vi "Music Visualizer Template LV2014.vi"() -> ()   [LabVIEW 2014]
uses:
  <vilib>/sound2/lvsound2.llb/Sampling Mode.ctl
  <vilib>/sound2/lvsound2.llb/Sound File Info (path).vi
  <vilib>/sound2/lvsound2.llb/Sound File Read Open.vi
  <vilib>/sound2/lvsound2.llb/Sound File Read (DBL).vi
  <vilib>/sound2/lvsound2.llb/Sound Output Write (DBL).vi
panel:
  in  "Stop":bool
  in  "Buffer Size (samples)":i32=2048
  in  "Music File":path
  # "Your visualizer here."
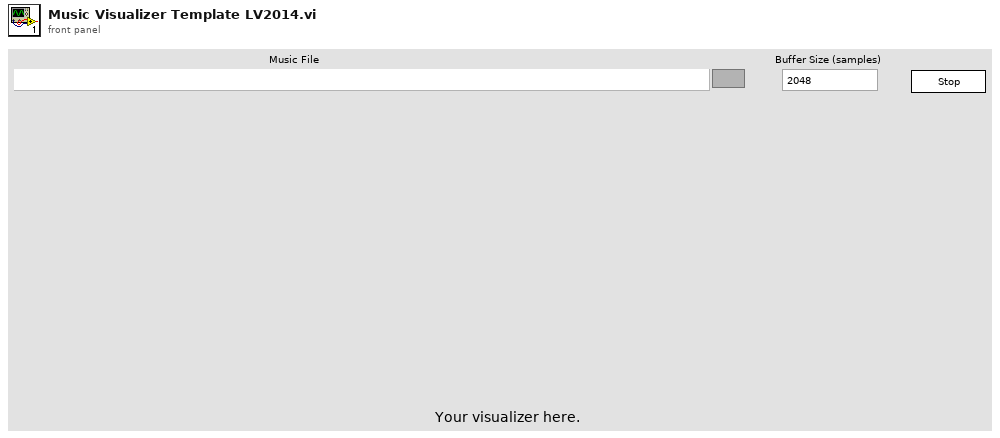
[diagram p1: front panel]
types:
  T1 = typedef "Sampling Mode.ctl" = i32
  T2 = typedef "Sound Data Format.ctl" = cluster{"sample rate (S/s)":dbl, "number of channels":i32, "bits per sample":i32}
  T3 = typedef "Sound Output Task ID.ctl" = u32
  T4 = typedef "Sound File Refnum.ctl" = refnum<file>
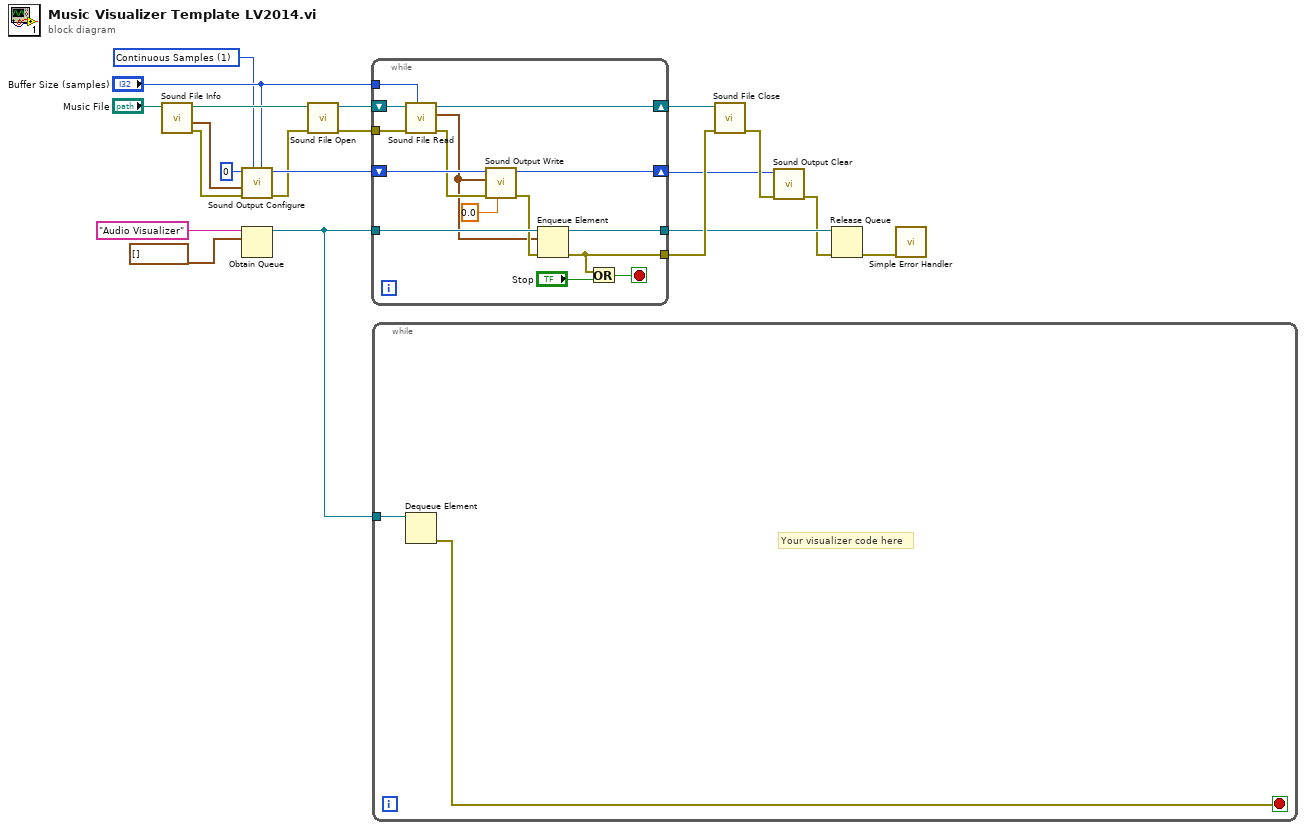
[diagram p0: block diagram]
diagram:
  w1 = T1 1 items=["Finite Samples", "Continuous Samples"] ("sample mode")
  n1 = call-poly <vilib>:"Sound File Info.vi"("path"="Music File") -> ("error out"=w4:errorcluster, "sound format"=w11:T2, "path out"=w14:path)  [unwired: 7 in, 1 out]
  n2 = call <vilib>:"Sound Output Configure.vi"("number of samples/ch"="Buffer Size (samples)", "sample mode"=w1, "error in (no error)"=w4, "sound format"=w11, "device ID"=u32 0) -> ("error out"=w3:errorcluster, "task ID"=w9:T3)  [unwired: 5 in]
  n3 = Obtain Queue(name (unnamed)="Audio Visualizer", element data type=waveform(dbl)[] [] ("data")) -> (queue out=w8:refnum<queue>)  [unwired: 3 in, 2 out]
  n4 = call-poly <vilib>:"Sound File Open.vi"("error in (no error)"=w3, "path"=w14) -> ("error out"=w19:errorcluster, "sound file refnum"=w21:T4)  [unwired: 8 in]
  n5 = while {
    tunnel: "Buffer Size (samples)" -> [w35]
    shift-right: [w34] -> w20
    shift-left: w21 -> [w36]
    tunnel: w19 -> [w33]
    tunnel: [w29] -> w18
    tunnel: w8 -> [w30]
    tunnel: [w28] -> w17
    shift-right: [w24] -> w5
    shift-left: w9 -> [w27]
    stop <- w32 stop-if-true
    n6 = call-poly <vilib>:"Sound File Read.vi"("number of samples/ch (-1: all)"=w35, "error in (no error)"=w33, "sound file refnum"=w36) -> ("error out"=w26:errorcluster, "data"=w23:waveform(dbl)[], "sound file refnum out"=w34:T4)  [unwired: 4 in, 2 out]
    n7 = call-poly <vilib>:"Sound Output Write.vi"("timeout (sec)"=0.0, "error in (no error)"=w26, "data"=w23, "task ID"=w27) -> ("error out"=w25:errorcluster, "task ID out"=w24:T3)  [unwired: 6 in]
    n8 = Enqueue Element(queue=w30, element=w23, error in (no error)=w25) -> (queue out=w28:refnum<queue>, error out=w29:errorcluster)  [unwired: 1 in, 1 out]
    n9 = Or(x=w29, y="Stop") -> (x .or. y?=w32:bool)
  }
  n10 = while {
    tunnel: w8 -> [w38]
    stop <- w37 stop-if-true
    # "Your visualizer code here"
    n11 = Dequeue Element(queue=w38) -> (error out=w37:errorcluster)  [unwired: 2 in, 3 out]
  }
  n12 = call <vilib>:"Sound File Close.vi"("error in (no error)"=w18, "sound file refnum"=w20) -> ("error out"=w7:errorcluster)  [unwired: 9 in]
  n13 = call <vilib>:"Sound Output Clear.vi"("error in (no error)"=w7, "task ID"=w5) -> ("error out"=w6:errorcluster)  [unwired: 9 in]
  n14 = Release Queue(queue=w17, error in (no error)=w6) -> (error out=w16:errorcluster)  [unwired: 1 in, 2 out]
  n15 = call <vilib>:"Simple Error Handler.vi"("error in (no error)"=w16) -> ()  [unwired: 4 in, 5 out]
